vi "ExtendedKalmanFilter_Correct.vi"(4 "H_FuncExtra":variant, 6 "H_Func":T1, 7 "Rows":i32, 8 "R":T2, 9 "Y":T2, 10 "U":T2, 11 "in ExtendedKalmanFiilter":T3) -> (0 "Error":bool, 3 "out ExtendedKalmanFiilter":T3)   [LabVIEW 2019, in "Trajectory_Library.lvlib"]
doc: "Creates a new LINEAR SYSTEM data cluster with the specified values. \n\n\nInputs: \n - XXX -- XXX.\n\nOutputs:\n - XXX -- XXX."
uses:
  Trajectory_Library.lvlib
  EXTENDED_KALMAN_FILTER.ctl
  <vilib>/Analysis/Matrix/Datatypes/RealMatrix.ctl
  BiFun_Matrix_FUNC_TYPE.ctl
  <vilib>/Analysis/7linalg.llb/Real Transpose Matrix.vi
  <vilib>/Analysis/baseanly.llb/Real A x B.vi
  MatBuilder_Create.vi
  <vilib>/Analysis/7linalg.llb/Create Special Matrix.vi
  <vilib>/Analysis/7linalg.llb/Create Special Real Matrix.vi
  <vilib>/Analysis/Matrix/Numeric/Subtract/Subtract - RM,RM.vi
  <vilib>/Analysis/Matrix/Numeric/Add/Add - RM,RM.vi
  <vilib>/Analysis/7linalg.llb/Solve Linear Equations (multiple right hand).vi
  <vilib>/Analysis/Matrix/NI_Matrix.lvlib
  <vilib>/Analysis/NI_AALPro.lvlib
  <vilib>/Analysis/NI_AALBase.lvlib
panel:
  # "<Inputs, 1>"
  # "<Rows, 1>"
  # "<Rows, Rows>"
  # "State Estimate <Statess,1>"
  # "<States, States>"
  # "<States, States>"
  # "<Statess,  States>"
  # "<Outputs, Outputs>"
  # "State Estimate <Statess,1>"
  # "<States, States>"
  # "<States, States>"
  # "<Statess,  States>"
  # "<Outputs, Outputs>"
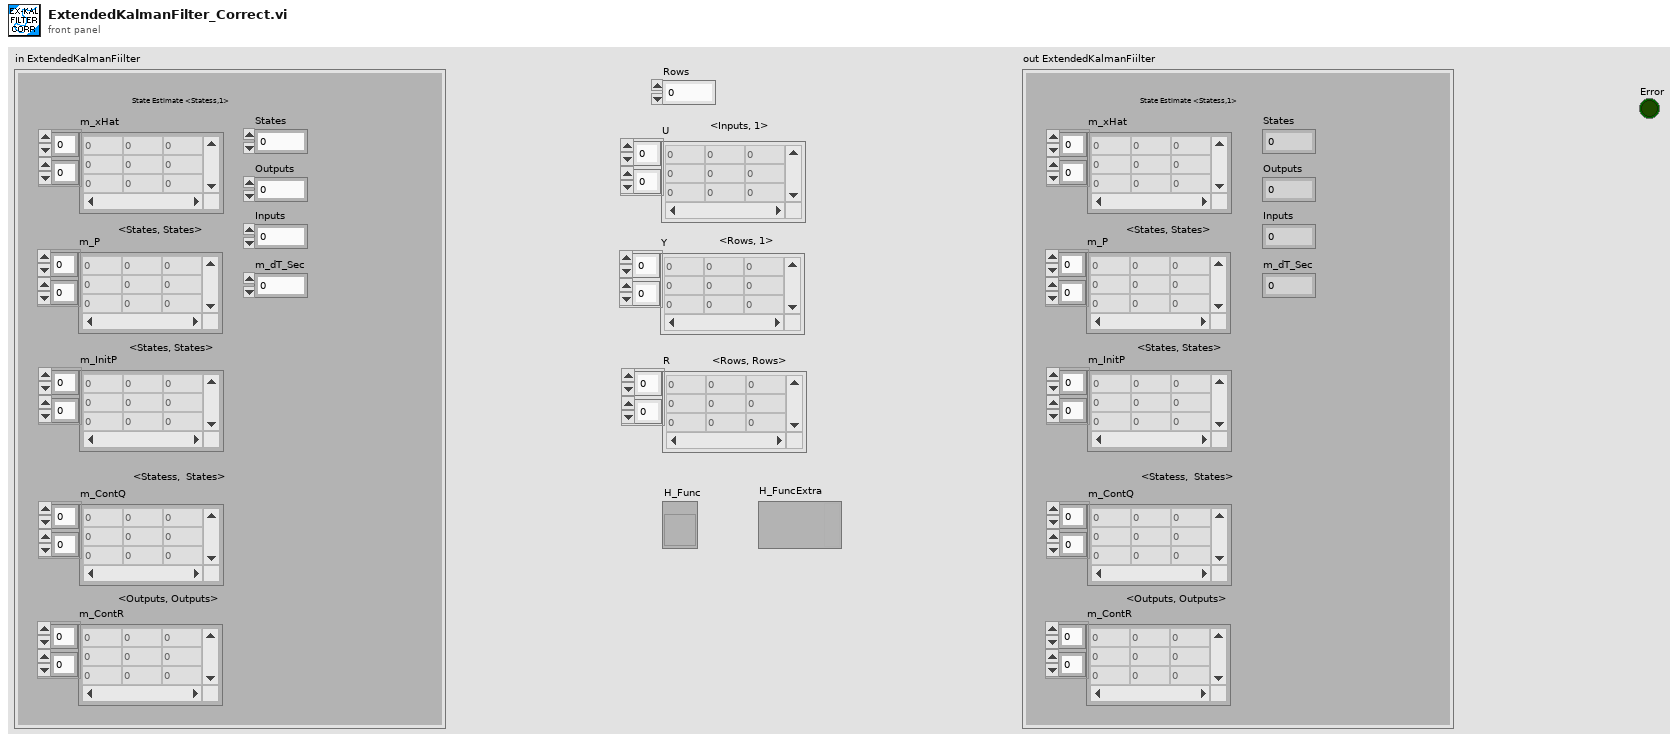
[diagram p1: front panel]
types:
  T1 = typedef "Trajectory_Library.lvlib/BiFun_Matrix_FUNC_TYPE.ctl" = refnum<vi>
  T2 = typedef "NI_Matrix.lvlib/RealMatrix.ctl" = dbl[][]
  T3 = typedef "Trajectory_Library.lvlib/EXTENDED_KALMAN_FILTER.ctl" = cluster{"m_P":T2, "m_xHat":T2, "States":i32, "Outputs":i32, "m_ContR":T2, "m_ContQ":T2, "m_dT_Sec":dbl, "Inputs":i32, "m_InitP":T2}
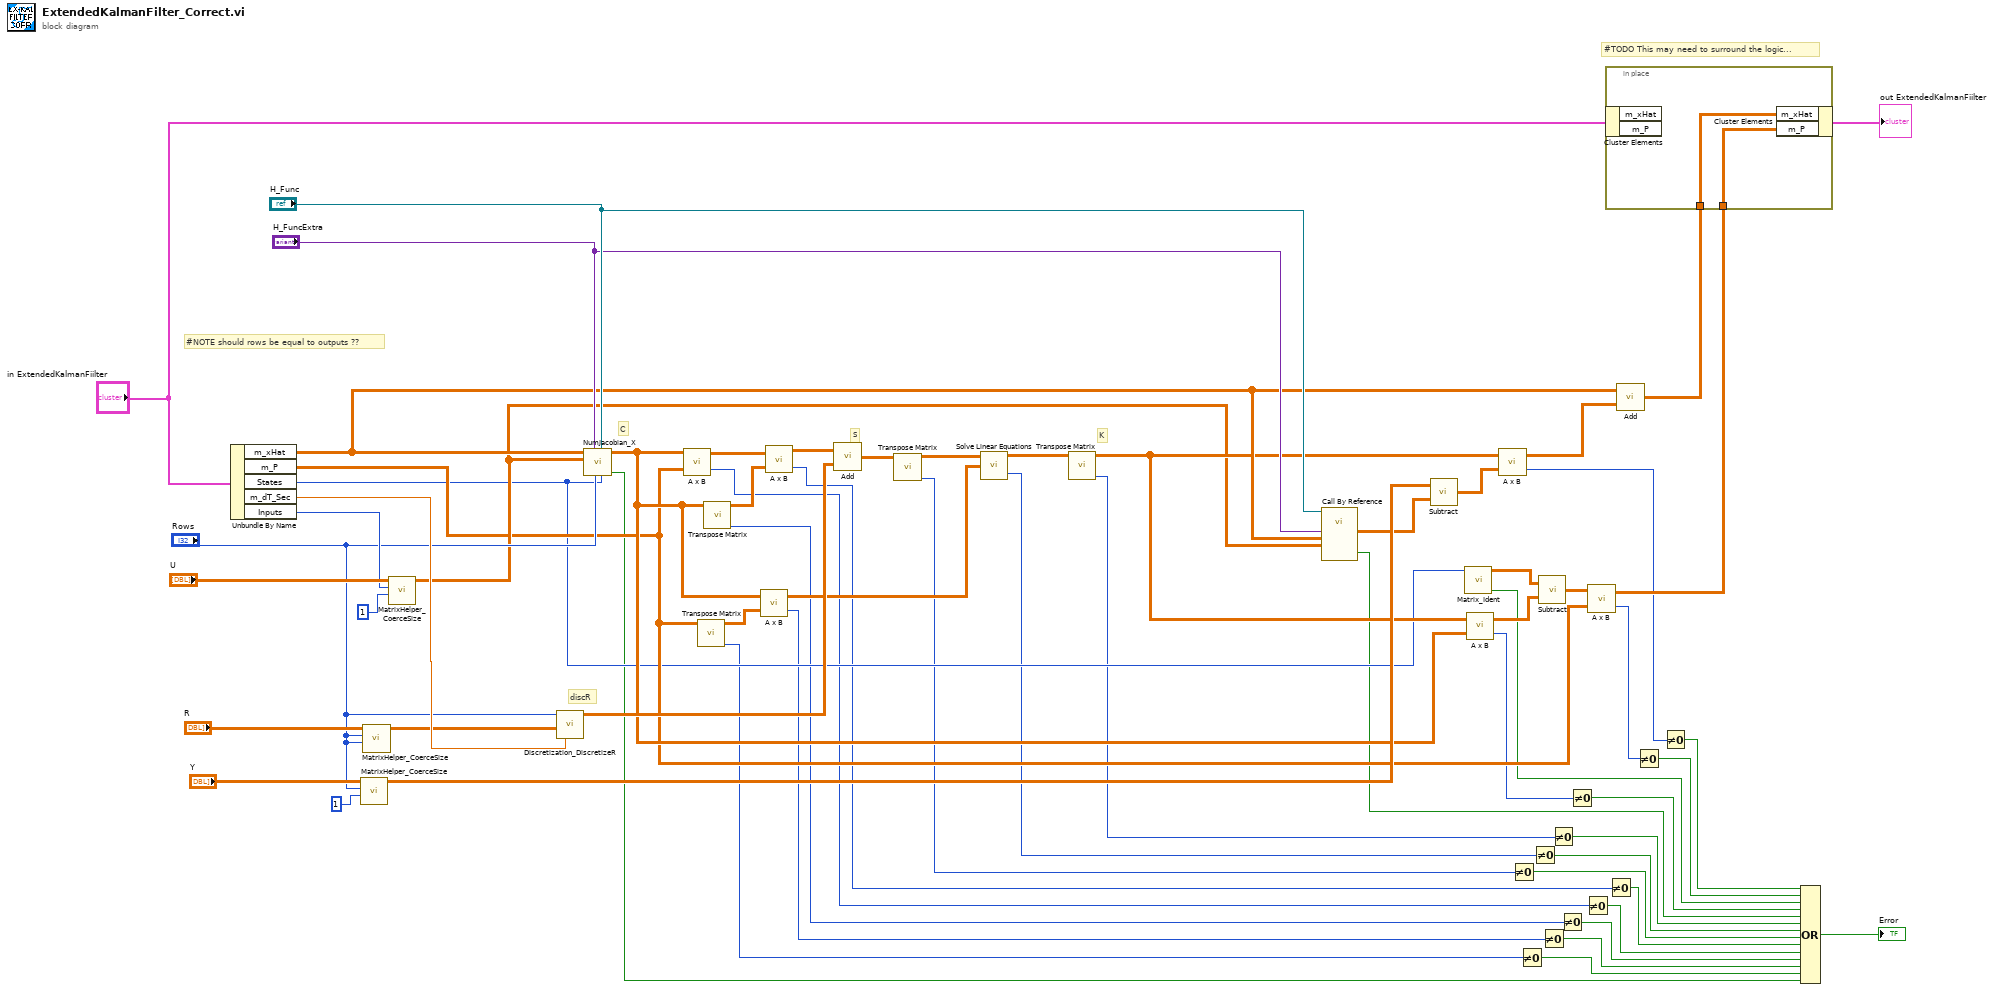
[diagram p0: block diagram]
diagram:
  # "K"
  # "S"
  # "C"
  # "#NOTE should rows be equal to outputs ??"
  # "#TODO This may need to surround the logic..."
  # "discR"
  n1 = Unbundle By Name("in ExtendedKalmanFiilter") -> ("m_xHat"=w35:T2, "m_P"=w25:T2, "States"=w24:i32, "m_dT_Sec"=w61:dbl, "Inputs"=w54:i32)
  n2 = call "MatrixHelper_CoerceSize.vi"("Columns"=1, "Rows"="Rows", "input matrix"="Y") -> ("output matrix"=w37:T2)  [unwired: 8 in]
  n3 = call "MatrixHelper_CoerceSize.vi"("Columns"="Rows", "Rows"="Rows", "input matrix"="R") -> ("output matrix"=w50:T2)  [unwired: 8 in]
  n4 = call "MatrixHelper_CoerceSize.vi"("Columns"=1, "Rows"=w54, "input matrix"="U") -> ("output matrix"=w26:T2)  [unwired: 8 in]
  n5 = call "Discretization_DiscretizeR.vi"("dT_Seconds"=w61, "ContR"=w50, "Outputs"="Rows") -> ("DiscR"=w42:T2)  [unwired: 8 in]
  n6 = call "NumJacobian_X.vi"("States"=w24, "F_FUNC"="H_Func", "Rows"="Rows", "ExtraPassedData"="H_FuncExtra", "U"=w26, "X"=w35) -> ("Error"=w22:bool, "Result"=w30:T2)  [unwired: 4 in]
  n7 = call-poly <vilib>:"A x B.vi"("B"=w25, "A"=w30) -> ("error"=w17:i32, "A x B"=w45:T2)
  n8 = call-poly <vilib>:"Transpose Matrix.vi"("Input Matrix"=w25) -> ("error"=w21:i32, "Matrix Transpose"=w48:T2)  [unwired: 9 in]
  n9 = call-poly <vilib>:"Transpose Matrix.vi"("Input Matrix"=w30) -> ("error"=w19:i32, "Matrix Transpose"=w44:T2)  [unwired: 9 in]
  n10 = call-poly <vilib>:"A x B.vi"("B"=w48, "A"=w30) -> ("error"=w20:i32, "A x B"=w39:T2)
  n11 = call-poly <vilib>:"A x B.vi"("B"=w44, "A"=w45) -> ("error"=w16:i32, "A x B"=w43:T2)
  n12 = call-poly <vilib>:"Add.vi"("Real Matrix B"=w42, "Real Matrix A"=w43) -> ("A + B"=w41:T2)
  n13 = call-poly <vilib>:"Transpose Matrix.vi"("Input Matrix"=w41) -> ("error"=w15:i32, "Matrix Transpose"=w40:T2)  [unwired: 9 in]
  n14 = call-poly <vilib>:"Solve Linear Equations.vi"("Known Matrix"=w39, "Input Matrix"=w40) -> ("error"=w14:i32, "Solution Matrix"=w38:T2)  [unwired: 1 in]
  n15 = call-poly <vilib>:"Transpose Matrix.vi"("Input Matrix"=w38) -> ("error"=w13:i32, "Matrix Transpose"=w31:T2)  [unwired: 9 in]
  n16 = call-by-ref "?"(reference="H_Func", "U"=w26, "X"=w35, "Variant"="H_FuncExtra") -> ("Error"=w8:bool, "NewX"=w36:T2)  [unwired: 8 in, 2 out]
  n17 = call-poly <vilib>:"Subtract.vi"("Real Matrix B"=w36, "Real Matrix A"=w37) -> ("A - B"=w32:T2)
  n18 = call "Matrix_Ident.vi"("Size"=w24) -> ("Error"=w5:bool, "output matrix"=w29:T2)  [unwired: 9 in]
  n19 = call-poly <vilib>:"A x B.vi"("B"=w30, "A"=w31) -> ("error"=w7:i32, "A x B"=w28:T2)
  n20 = call-poly <vilib>:"A x B.vi"("B"=w32, "A"=w31) -> ("error"=w2:i32, "A x B"=w34:T2)
  n21 = Not Equal To 0?(x=w15) -> (x != 0?=w11:bool)
  n22 = Not Equal To 0?(x=w21) -> (x != 0?=w60:bool)
  n23 = Not Equal To 0?(x=w14) -> (x != 0?=w10:bool)
  n24 = call-poly <vilib>:"Subtract.vi"("Real Matrix B"=w28, "Real Matrix A"=w29) -> ("A - B"=w27:T2)
  n25 = Not Equal To 0?(x=w20) -> (x != 0?=w59:bool)
  n26 = Not Equal To 0?(x=w13) -> (x != 0?=w9:bool)
  n27 = Not Equal To 0?(x=w19) -> (x != 0?=w58:bool)
  n28 = Not Equal To 0?(x=w7) -> (x != 0?=w6:bool)
  n29 = Not Equal To 0?(x=w17) -> (x != 0?=w18:bool)
  n30 = call-poly <vilib>:"A x B.vi"("B"=w25, "A"=w27) -> ("error"=w4:i32, "A x B"=w23:T2)
  n31 = Not Equal To 0?(x=w16) -> (x != 0?=w12:bool)
  n32 = call-poly <vilib>:"Add.vi"("Real Matrix B"=w34, "Real Matrix A"=w35) -> ("A + B"=w33:T2)
  n33 = in-place {
    in-place-border: w23 -> [w65]
    in-place-border: w33 -> [w64]
    n34 = in-place-cluster #1("in ExtendedKalmanFiilter") -> ()  [unwired: 2 out]
    n35 = in-place-cluster #1("m_xHat"=w64, "m_P"=w65) -> (→"out ExtendedKalmanFiilter":T3)
  }
  n36 = Not Equal To 0?(x=w4) -> (x != 0?=w3:bool)
  n37 = Not Equal To 0?(x=w2) -> (x != 0?=w1:bool)
  n38 = Compound Arithmetic op=OR(w1, w3, w5, w6, w8, w9, w10, w11, w12, w18, w58, w59, w60, w22) -> (→"Error":bool)
